vi "Check Control.vi"(8 "error in (no error)":errorcluster, 10 "Control":refnum<vi>, 11 "Search in":refnum<class "Search.lvclass">) -> (0 "error out":errorcluster, 2 "Match?":bool, 3 "Search out":refnum<class "Search.lvclass">)   [LabVIEW 2020, in "Better Search.lvlib" / "Search.lvclass"]
uses:
  Search.lvclass
  Search.lvclass/Search.ctl
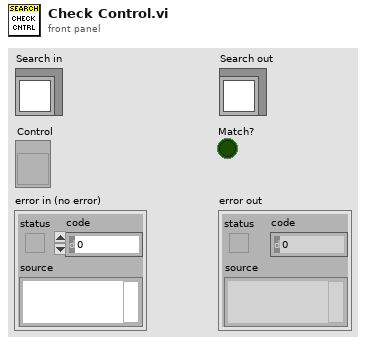
[diagram p1: front panel]
types:
  T1 = typedef "Better Search.lvlib/Search Type.ctl" = enum16{"Generic", "Text", "Data Type", "VI", "Node"}
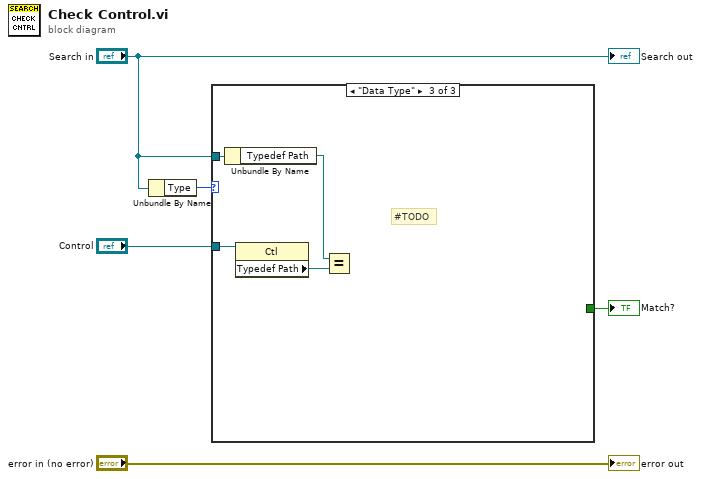
[diagram p0: block diagram]
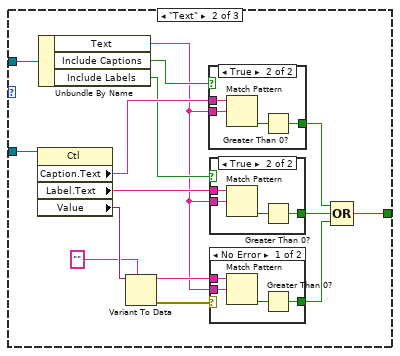
[diagram p3: hidden frame]
diagram:
  n1 = Unbundle By Name("Search in") -> ("Type"=w1:T1)
  n2 = case shown="\"Data Type\"" w1 {
    tunnel: [_ w13 _] -> w4
    tunnel: "Control" -> [_ w12 w36]
    tunnel: "Search in" -> [_ w6 w35]
    frame Default {
    }
    frame "Text" {
      n3 = property class="Ctl"(reference=w12) -> ("Caption.Text"=w15:string, "Label.Text"=w16:string, "Value"=w20:variant)  [unwired: 1 in, 2 out]
      n4 = Unbundle By Name(w6) -> ("Text"=w7:string, "Include Captions"=w9:bool, "Include Labels"=w8:bool)
      n5 = Variant To Data(type="", Variant=w20) -> (data=w17:string, error out=w18:errorcluster)  [unwired: 1 in]
      n6 = case shown="True" w9 {
        tunnel: w15 -> [_ w28]
        tunnel: [_ w26] -> w10
        tunnel: w7 -> [_ w25]
        frame False {
        }
        frame True {
          n7 = Match Pattern(string=w28, regular expression=w25) -> (offset past match=w27:i32)  [unwired: 1 in, 3 out]
          n8 = Greater Than 0?(x=w27) -> (x > 0?=w26:bool)
        }
      }
      n9 = case shown="True" w8 {
        tunnel: w16 -> [_ w24]
        tunnel: [_ w22] -> w11
        tunnel: w7 -> [_ w21]
        frame False {
        }
        frame True {
          n10 = Match Pattern(string=w24, regular expression=w21) -> (offset past match=w23:i32)  [unwired: 1 in, 3 out]
          n11 = Greater Than 0?(x=w23) -> (x > 0?=w22:bool)
        }
      }
      n12 = case shown="No Error" w18 {
        tunnel: w17 -> [w32 _]
        tunnel: [w30 _] -> w14
        tunnel: w7 -> [w29 _]
        frame No Error {
          n13 = Match Pattern(string=w32, regular expression=w29) -> (offset past match=w31:i32)  [unwired: 1 in, 3 out]
          n14 = Greater Than 0?(x=w31) -> (x > 0?=w30:bool)
        }
        frame Error {
        }
      }
      n15 = Compound Arithmetic op=OR(w10, w11, w14) -> (w13:bool)
    }
    frame "Data Type" {
      # "#TODO"
      n16 = Unbundle By Name(w35) -> ("Typedef Path"=w33:path)
      n17 = property class="Ctl"(reference=w36) -> ("Typedef Path"=w34:path)  [unwired: 1 in, 2 out]
      n18 = Equal?(x=w33, y=w34) -> ()  [unwired: 1 out]
    }
  }
  "Match?" <- w4
  "error out" <- "error in (no error)"
  "Search out" <- "Search in"
